vi "Publish ILC Outputs.vi"(8 "error in (no error)":errorcluster, 11 "Model in":refnum<class "Model.lvclass">) -> (0 "error out":errorcluster, 3 "Model out":refnum<class "Model.lvclass">)   [LabVIEW 2015, in "Model.lvclass"]
uses:
  Model.lvclass
  Typedefs/ILC ADC.ctl
  Model.lvclass/Model.ctl
  <userlib>/Common/ILC/ILC/ILC.lvclass/ILC.ctl
  UserEvents/UserEvents.lvclass/UserEvents.ctl
  UserEvents/UserEvents.lvclass
  <userlib>/Common/ILC/ILC/ILC.lvclass
  View/FAMT Views.lvlib
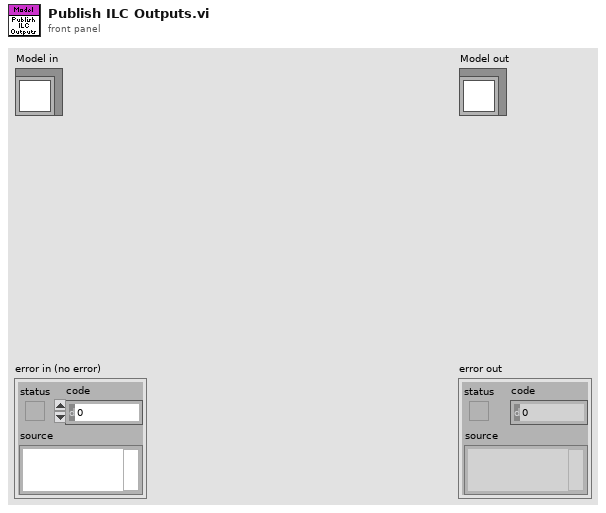
[diagram p1: front panel]
types:
  T1 = typedef "FAMT Views.lvlib/ILC ADC.ctl" = cluster{"Ch1":dbl[unit], "Ch2":dbl[unit], "Ch3":dbl[unit], "Ch4":dbl[unit]}
  T2 = typedef "ILCCommon.lvlib/ILCTypedefs.lvlib/ADC Eng.ctl" = cluster{"Ch1":dbl[unit], "Ch2":dbl[unit], "Ch3":dbl[unit], "Ch4":dbl[unit]}
  T3 = typedef "FAMT Typedefs.lvlib/Publish Data Events.ctl" = cluster{"State":refnum<user-event>, "ErrorCode":refnum<user-event>, "FC1 ILC Outputs":refnum<user-event>, "LogPath":refnum<user-event>, "ILC Inputs":refnum<user-event>, "Scan Progress":refnum<user-event>, "FC2 ILC Outputs":refnum<user-event>}
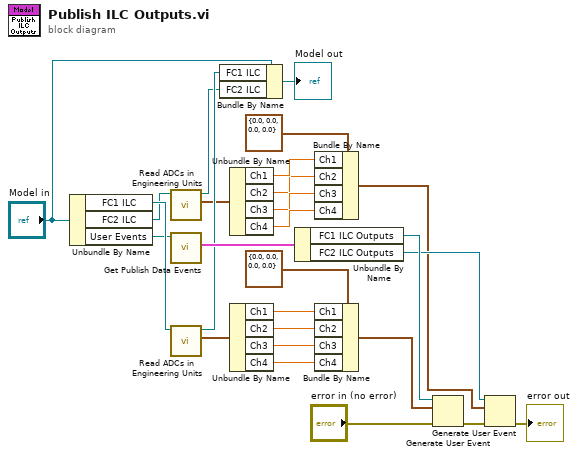
[diagram p0: block diagram]
diagram:
  n1 = Unbundle By Name("Model in") -> ("FC1 ILC"=w26:refnum<class "ILC.lvclass">, "FC2 ILC"=w12:refnum<class "ILC.lvclass">, "User Events"=w13:refnum<class "UserEvents.lvclass">)
  n2 = call <userlib>:"Read ADCs in Engineering Units.vi"("ILC in"=w12) -> ("ADCs in Engineering Units"=w2:T2, "ILC out"=w1:refnum<class "ILC.lvclass">)  [unwired: 9 in]
  n3 = call "Get Publish Data Events.vi"("UserEvents in"=w13) -> ("Publish Data Events"=w27:T3)  [unwired: 9 in, 1 out]
  n4 = call <userlib>:"Read ADCs in Engineering Units.vi"("ILC in"=w26) -> ("ADCs in Engineering Units"=w24:T2, "ILC out"=w17:refnum<class "ILC.lvclass">)  [unwired: 9 in]
  n5 = Bundle By Name(cluster="Model in", "FC1 ILC"=w17, "FC2 ILC"=w1) -> (→"Model out":refnum<class "Model.lvclass">)
  n6 = Unbundle By Name(w2) -> ("Ch1"=w11:dbl[unit], "Ch2"=w8:dbl[unit], "Ch3"=w9:dbl[unit], "Ch4"=w10:dbl[unit])
  n7 = Unbundle By Name(w24) -> ("Ch1"=w15:dbl[unit], "Ch2"=w23:dbl[unit], "Ch3"=w22:dbl[unit], "Ch4"=w21:dbl[unit])
  n8 = Unbundle By Name(w27) -> ("FC1 ILC Outputs"=w20:refnum<user-event>, "FC2 ILC Outputs"=w6:refnum<user-event>)
  n9 = Bundle By Name(cluster=T1 {"Ch1"=0.0, "Ch2"=0.0, "Ch3"=0.0, "Ch4"=0.0} ("Output Data"), "Ch1"=w11, "Ch2"=w8, "Ch3"=w9, "Ch4"=w10) -> (w3:T1)
  n10 = Bundle By Name(cluster=T1 {"Ch1"=0.0, "Ch2"=0.0, "Ch3"=0.0, "Ch4"=0.0} ("Output Data"), "Ch1"=w15, "Ch2"=w23, "Ch3"=w22, "Ch4"=w21) -> (w19:T1)
  n11 = Generate User Event(user event=w20, event data cluster=w19, error in="error in (no error)") -> (error out=w5:errorcluster)  [unwired: 1 in, 1 out]
  n12 = Generate User Event(user event=w6, event data cluster=w3, error in=w5) -> (error out=→"error out":errorcluster)  [unwired: 1 in, 1 out]
